vi "StreamEngine.Main.Stream.Stop.vi"(8 "error in (no error)":errorcluster, 9 "Exit?":bool, 10 "Stream.Qs.SubProcesses":T1, 11 "Stream Ref":T2) -> (0 "error out":errorcluster)   [LabVIEW 2025, in "XNET Bus Monitor Client.lvlib"]
uses:
  XNET Bus Monitor Client.lvlib
  xnet_can_bus_monitor_api_client/xnet_can_bus_monitor_api_client.lvlib
  Types/SubProcessEngine.CmdQueueData.ctl
  Types/SubProcessEngine.CmdQueueData.Cmd.ctl
  <vilib>/gRPC/LabVIEW gRPC Library/Shared/grpcId.ctl
  <vilib>/gRPC/LabVIEW gRPC Library/grpc-lvsupport-release.lvlib
  Types/SubProcessEngine.QueueRefs.ctl
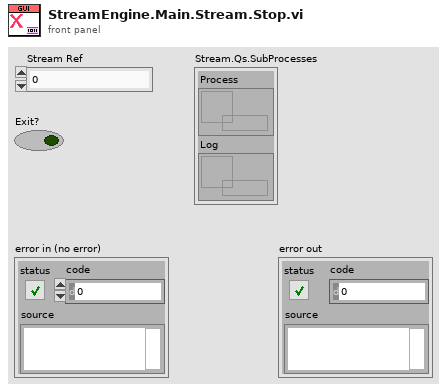
[diagram p1: front panel]
types:
  T1 = typedef "XNET Bus Monitor Client.lvlib/SubProcessEngine.QueueRefs.ctl" = cluster{"Process":refnum<queue>, "Log":refnum<queue>}
  T2 = typedef "grpc-lvsupport-release.lvlib/grpcId.ctl" = u64
  T3 = typedef "XNET Bus Monitor Client.lvlib/SubProcessEngine.CmdQueueData.Cmd.ctl" = enum16{"Arm", "Publish", "Stop", "Exit"}
  T4 = typedef "XNET Bus Monitor Client.lvlib/SubProcessEngine.CmdQueueData.ctl" = cluster{"Cmd":T3, "Parameters":variant}
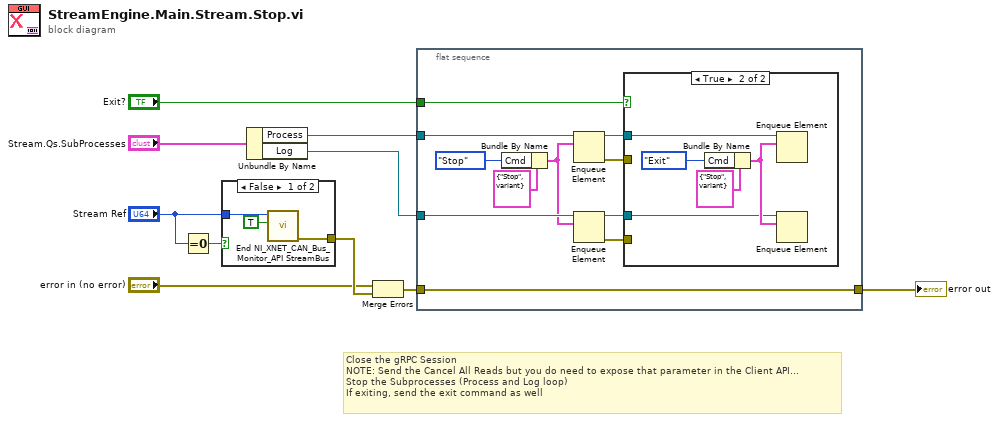
[diagram p0: block diagram]
diagram:
  # "Close the gRPC Session\nNOTE: Send the Cancel All Reads but you do need to expose that parameter in the Client API...\nStop the Subprocesses (Process and Log loop)\nIf exiting, send the exit command as well"
  n1 = Equal To 0?(x="Stream Ref") -> (x = 0?=w8:bool)
  n2 = case shown="False" w8 {
    tunnel: [w11 _] -> w10
    tunnel: "Stream Ref" -> [w13 _]
    frame False {
      n3 = call "End NI_XNET_CAN_Bus_Monitor_API StreamBus.vi"("Cancel All Reads (F)"=TRUE, "Call ID in"=w13) -> ("error out"=w11:errorcluster)  [unwired: 8 in, 1 out]
    }
    frame True {
    }
  }
  n4 = Unbundle By Name("Stream.Qs.SubProcesses") -> ("Process"=w3:refnum<queue>, "Log"=w2:refnum<queue>)
  n5 = Merge Errors("error in (no error)", w10) -> (w6:errorcluster)
  n6 = flat-sequence {
    tunnel: w6 -> [w24]
    tunnel: [w24] -> w5
    tunnel: w3 -> [w23]
    tunnel: w2 -> [w22]
    tunnel: "Exit?" -> [w16]
    frame #0 {
      n7 = Bundle By Name(cluster=T4 {"Cmd"=enum."Stop", "Parameters"=variant} ("element"), "Cmd"=SubProcessEngine.CmdQueueData.Cmd."Stop") -> (w20:T4)
      n8 = Enqueue Element(queue=w23, element=w20) -> (queue out=w18:refnum<queue>, error out=w15:errorcluster)  [unwired: 2 in, 1 out]
      n9 = Enqueue Element(queue=w22, element=w20) -> (queue out=w17:refnum<queue>, error out=w14:errorcluster)  [unwired: 2 in, 1 out]
      n10 = case shown="True" w16 {
        tunnel: w18 -> [_ w27]
        tunnel: w17 -> [_ w26]
        tunnel: w15 -> [_ _]
        tunnel: w14 -> [_ _]
        frame False {
        }
        frame True {
          n11 = Bundle By Name(cluster=T4 {"Cmd"=enum."Stop", "Parameters"=variant} ("element"), "Cmd"=SubProcessEngine.CmdQueueData.Cmd."Exit") -> (w28:T4)
          n12 = Enqueue Element(queue=w27, element=w28) -> ()  [unwired: 2 in, 3 out]
          n13 = Enqueue Element(queue=w26, element=w28) -> ()  [unwired: 2 in, 3 out]
        }
      }
    }
  }
  "error out" <- w5
